vi "ConfirmConnectionAndErrorStates.vi"(8 "error in (no error)":errorcluster, 10 "Address":u8, 11 "VISA resource name":refnum<visa-resource-name>) -> (0 "error out":errorcluster, 1 "Raw Response":string, 2 "Value":dbl, 3 "VISA resource name out":refnum<visa-resource-name>)   [LabVIEW 2020, in "driver_flodx_rtd.lvlib"]
doc: "Confirms connection and displays error states with device by sending back n,0,0.00,errorcode"
uses:
  <instrlib>/RxnRover/FloDx RTD Driver/driver_flodx_rtd.lvlib
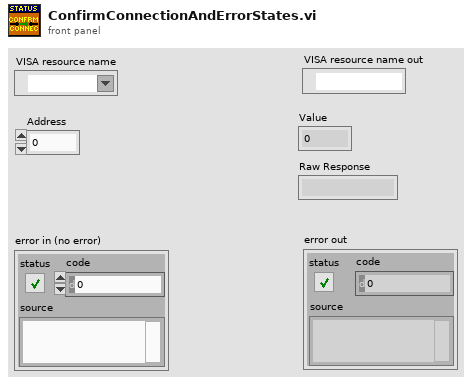
[diagram p1: front panel]
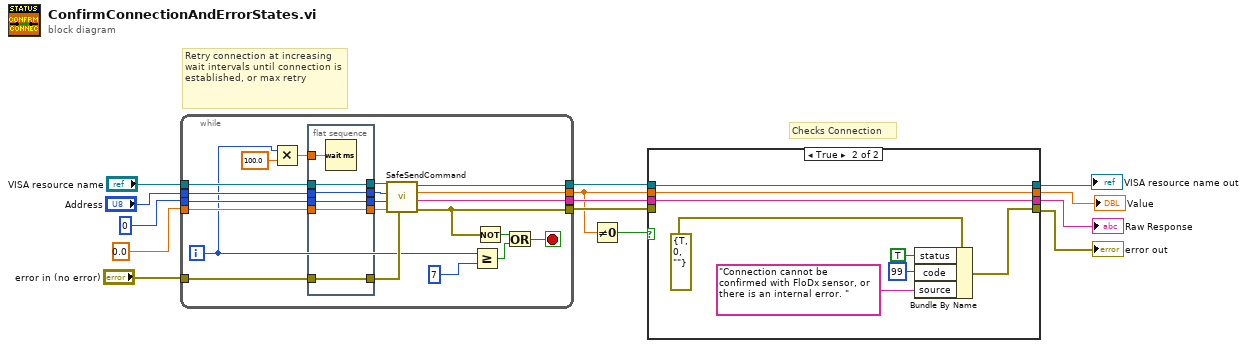
[diagram p0: block diagram]
diagram:
  # "Retry connection at increasing wait intervals until connection is established, or max retry"
  # "Checks Connection"
  n1 = while {
    tunnel: "Address" -> [w21]
    tunnel: u8 0 ("Command") -> [w23]
    tunnel: sgl 0.0 ("Parameter(float)") -> [w24]
    tunnel: [w34] -> w7
    tunnel: [w33] -> w5
    tunnel: "VISA resource name" -> [w18]
    tunnel: [w35] -> w9
    tunnel: "error in (no error)" -> [w26]
    tunnel: [w30] -> w8
    i -> [w15]
    stop <- w32 stop-if-true
    n2 = Multiply(x=w15, y=100.0) -> (x*y=w17:dbl)
    n3 = flat-sequence {
      tunnel: [w41] -> w27
      tunnel: w26 -> [w41]
      tunnel: [w40] -> w25
      tunnel: w24 -> [w40]
      tunnel: w23 -> [w39]
      tunnel: [w39] -> w22
      tunnel: w21 -> [w38]
      tunnel: [w38] -> w20
      tunnel: [w37] -> w19
      tunnel: w18 -> [w37]
      tunnel: w17 -> [w36]
      frame #0 {
        n4 = Wait (ms)(milliseconds to wait=w36) -> ()  [unwired: 1 out]
      }
    }
    n5 = call <instrlib>:"SafeSendCommand.vi"("error in"=w27, "Parameter"=w25, "Command #"=w22, "Address #"=w20, "VISA resource name"=w19) -> ("error out"=w30:errorcluster, "Raw Response"=w34:string, "Value"=w33:dbl, "VISA resource name out"=w35:refnum<visa-resource-name>)  [unwired: 3 in]
    n6 = Greater Or Equal?(x=w15, y=7) -> (x >= y?=w28:bool)
    n7 = Not(x=w30) -> (.not. x?=w31:bool)
    n8 = Or(x=w31, y=w28) -> (x .or. y?=w32:bool)
  }
  n9 = Not Equal To 0?(x=w5) -> (x != 0?=w6:bool)
  n10 = case shown="True" w6 {
    tunnel: [w44 w51] -> w3
    tunnel: [w45 w53] -> w1
    tunnel: w8 -> [w44 _]
    tunnel: w9 -> [w45 w53]
    tunnel: w5 -> [w43 w47]
    tunnel: w7 -> [w42 w46]
    tunnel: [w43 w47] -> w4
    tunnel: [w42 w46] -> w2
    frame False {
    }
    frame True {
      n11 = Bundle By Name(cluster=errorcluster {"status"=TRUE, "code"=0, "source"=""} ("error IO"), "status"=TRUE, "code"=99, "source"="Connection cannot be confirmed with FloDx sensor, or there is an internal error. ") -> (w51:errorcluster)
    }
  }
  "error out" <- w3
  "VISA resource name out" <- w1
  "Raw Response" <- w2
  "Value" <- w4
